vi "In Range.vi"(1 "Lower resistance (ohm)":dbl, 2 "Resistance (ohm)":dbl, 3 "Upper resistance (ohm)":dbl) -> (0 "range":enum16{"Lower", "In Range", "Greater"}(ring))   [LabVIEW 2018]
panel:
  out "greater?":bool
  out "lower?":bool
  out "in range?":bool
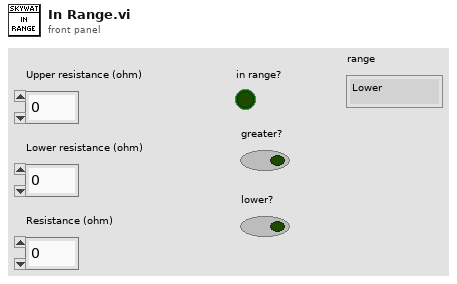
[diagram p1: front panel]
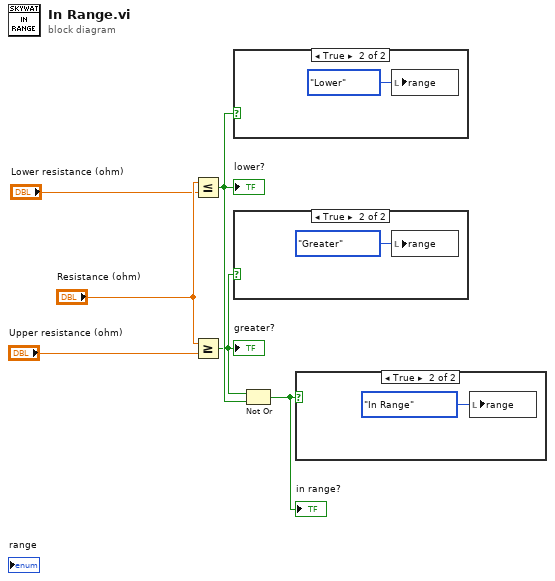
[diagram p0: block diagram]
diagram:
  n1 = Less Or Equal?(x="Resistance (ohm)", y="Lower resistance (ohm)") -> (x <= y?=w3:bool)
  "lower?" <- w3
  n2 = Greater Or Equal?(x="Resistance (ohm)", y="Upper resistance (ohm)") -> (x >= y?=w1:bool)
  "greater?" <- w1
  n3 = case shown="True" w3 {
    frame False {
    }
    frame True {
      n4 = local write "range"(enum16{"Lower", "In Range", "Greater"}."Lower" ("range")) -> ()
    }
  }
  n5 = case shown="True" w1 {
    frame False {
    }
    frame True {
      n6 = local write "range"(enum16{"Lower", "In Range", "Greater"}."Greater" ("range")) -> ()
    }
  }
  n7 = Not Or(1:w3, 2:w1) -> (0:w2:bool)
  "in range?" <- w2
  n8 = case shown="True" w2 {
    frame False {
    }
    frame True {
      n9 = local write "range"(enum16{"Lower", "In Range", "Greater"}."In Range" ("range")) -> ()
    }
  }
